vi "TestModule_Main.vi"() -> ()   [LabVIEW 2021]
uses:
  SubVI/TcpCmd_003/SubVI/SampleStatus.ctl
  SubVI/TcpCmd_003/SubVI/TcpCommunicationClientCMD.ctl
  SubVI/ErrorLogMode.ctl
  SubVI/MainStatus.ctl
panel:
  out "Message":string
  in  "SampleStatus":T1
  in  "Main Tab":enum32{"操作", "TCP"}(tab)
  out "TCPDataLog":T2(array[cluster])
  in  "Send Data":string
  in  "Send":bool
  out "ReadData":string
  in  "中央PCアドレス":string="192.168.0.1"
  in  "ポート":u16=8501
  out "TcpOK?":bool
  out "SettingFilePath":path
  in  "DataFilePath":path=path "Test_DataFile"
  out "SampleName":string
  in  "Quit":bool
  out "Quit?":bool
  # "Test Module Main"
  # "Ver. 0.01"
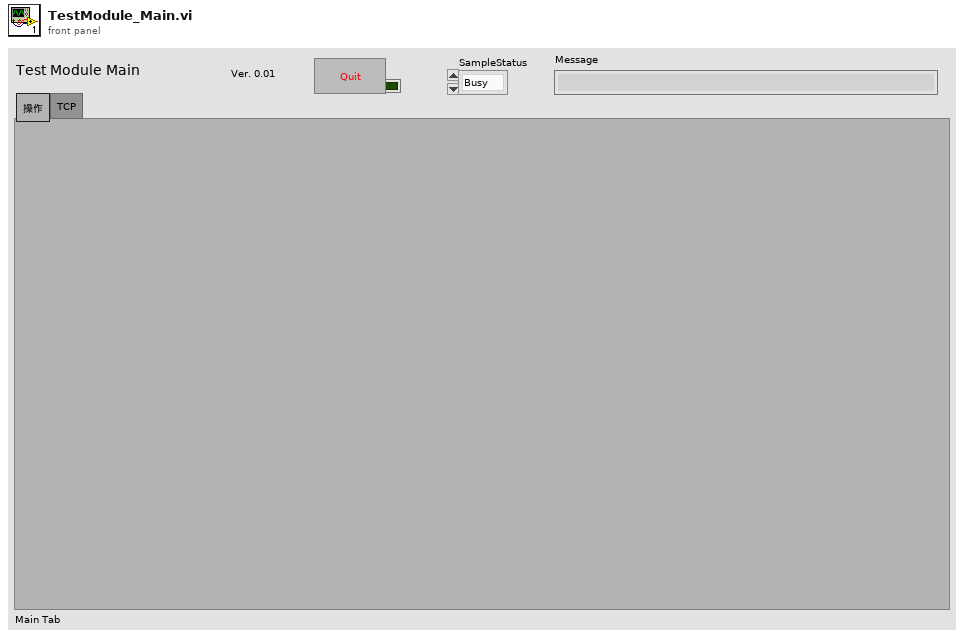
[diagram p1: front panel]
types:
  T1 = typedef "SampleStatus.ctl" = enum16{"Busy", "Ready", "Done", "Error"}
  T2 = cluster{"Command":string, "ReadData":string, "Send Data":string}[]
  T3 = typedef "TcpCommunicationClientCMD.ctl" = enum16{"Read", "Write", "Close"}
  T4 = typedef "ErrorLogMode.ctl" = enum16{"Init", "Add"}
  T5 = typedef "MainStatus.ctl" = enum16{"Init", "Status", "Placed", "Setting", "Start", "Data", "Collected", "Quit"}
  T6 = cluster{"Command":string, "ReadData":string, "t":string}
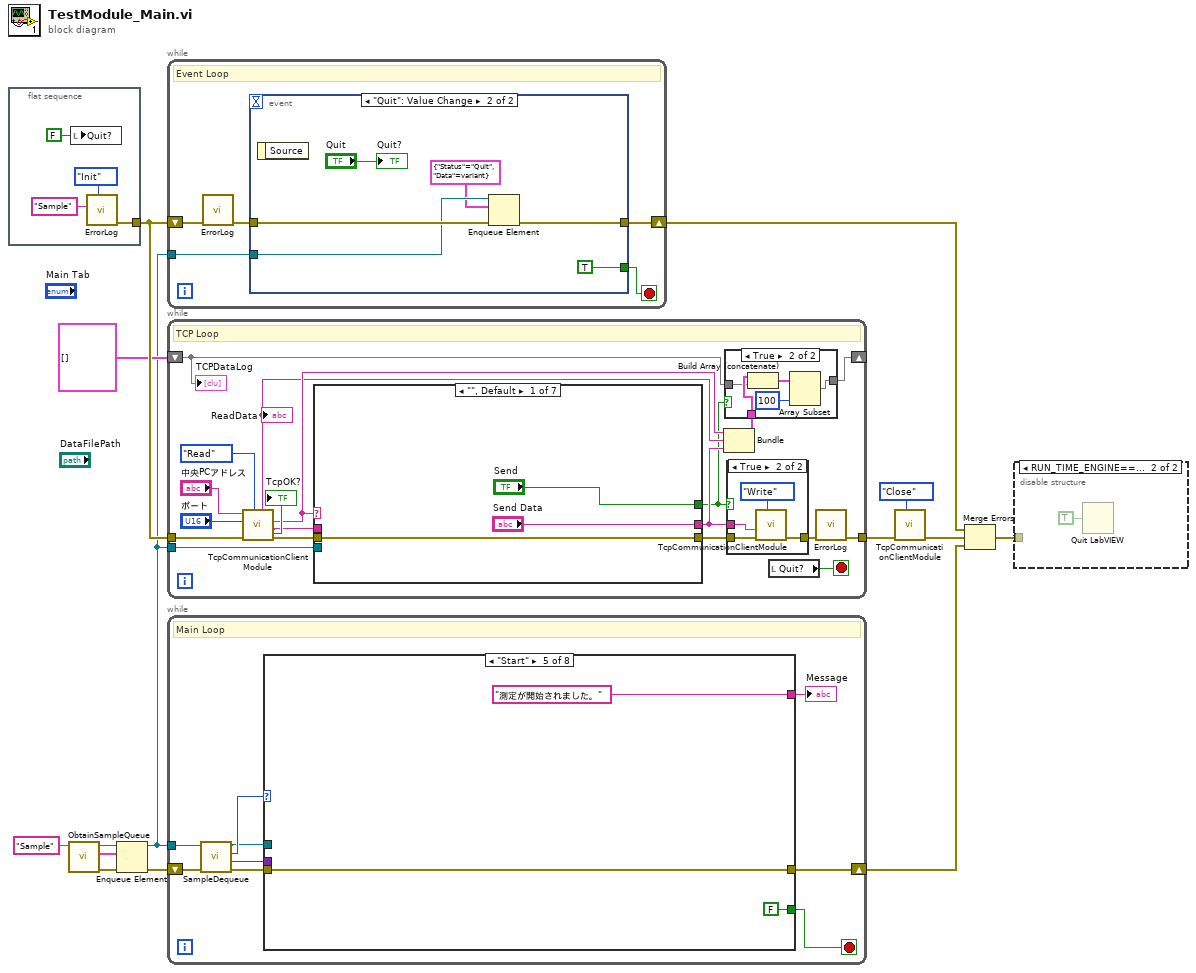
[diagram p0: block diagram]
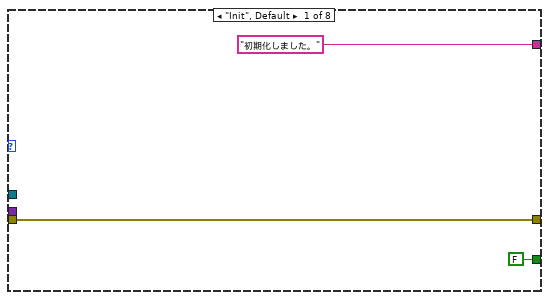
[diagram p3: hidden frame]
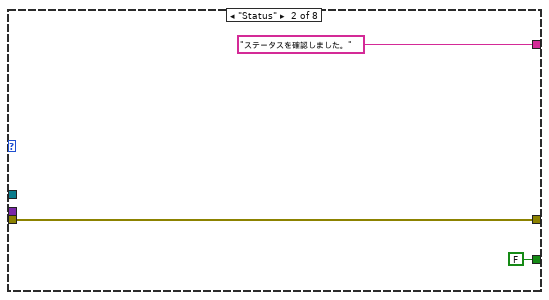
[diagram p4: hidden frame]
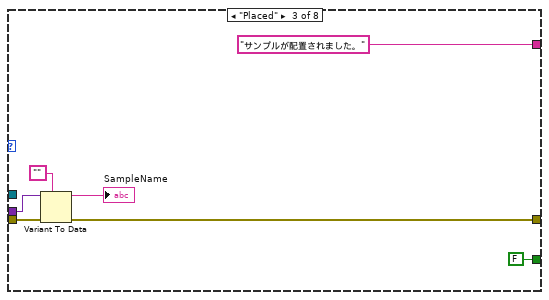
[diagram p5: hidden frame]
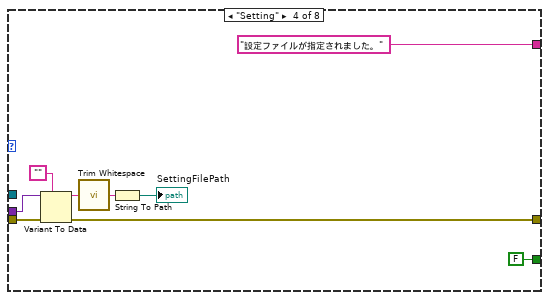
[diagram p6: hidden frame]
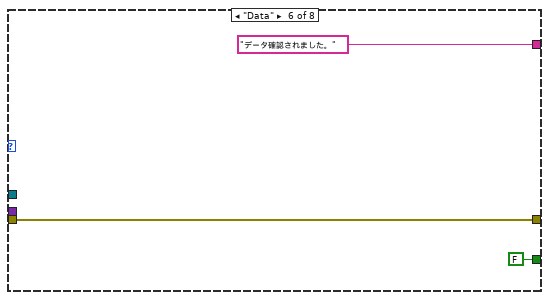
[diagram p7: hidden frame]
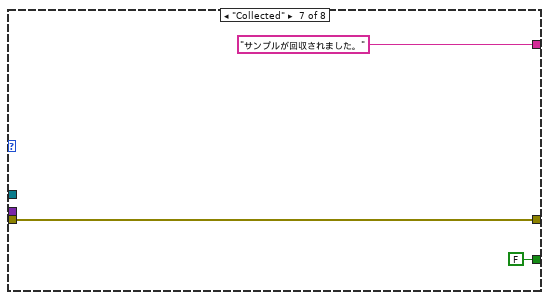
[diagram p8: hidden frame]
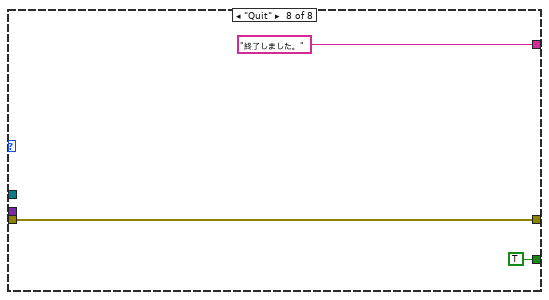
[diagram p9: hidden frame]
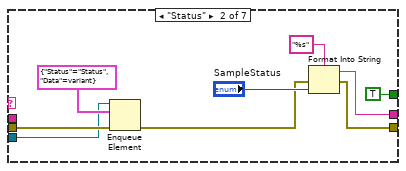
[diagram p12: hidden frame]
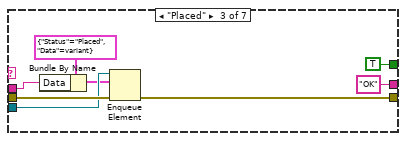
[diagram p13: hidden frame]
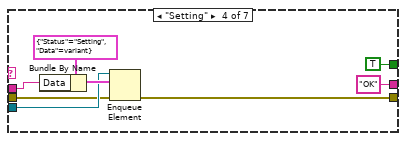
[diagram p14: hidden frame]
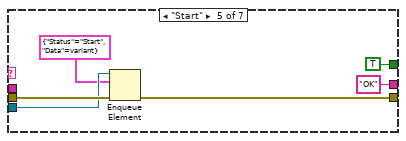
[diagram p15: hidden frame]
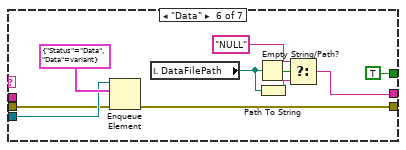
[diagram p16: hidden frame]
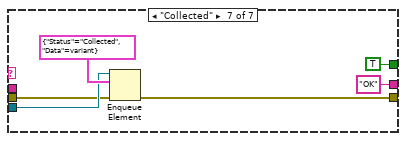
[diagram p17: hidden frame]
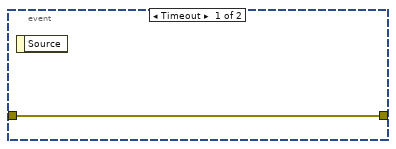
[diagram p18: hidden frame]
diagram:
  n1 = flat-sequence {
    tunnel: [w18] -> w14
    frame #0 {
      n2 = local write "Quit?"(FALSE ("Quit?")) -> ()
      n3 = call "ErrorLog.vi"("ErrorLogMode"=ErrorLogMode."Init", "ModuleName"="Sample") -> ("error out"=w18:errorcluster)  [unwired: 8 in, 1 out]
    }
  }
  n4 = call "ObtainSampleQueue.vi"("QName"="Sample") -> ("ErrorOut"=w10:errorcluster, "SampleQ"=w7:cluster{"Status":T5, "Data":variant}, "QueueOut"=w9:refnum<queue>)  [unwired: 8 in]
  n5 = Enqueue Element(queue=w9, element=w7, error in (no error)=w10) -> (queue out=w5:refnum<queue>, error out=w8:errorcluster)  [unwired: 1 in, 1 out]
  n6 = while {
    shift-right: [w21] -> w3
    shift-left: w14 -> [w22]
    tunnel: w5 -> [w19]
    stop <- w23 stop-if-true
    # "Event Loop"
    n7 = call "ErrorLog.vi"("error in (no error)"=w22) -> ("error out"=w20:errorcluster)  [unwired: 9 in, 1 out]
    n8 = event shown="[1] \"Quit\": Value Change" {
      selector: _ -> [_ _]
      dyn-events: _ -> [_ _]
      timeout: _ -> [_ _]
      tunnel: [_ TRUE] -> w23
      tunnel: [w24 w27] -> w21
      tunnel: w20 -> [w24 w28]
      tunnel: w19 -> [_ w26]
      event Timeout {
        n9 = event-data() -> ()  [unwired: 1 in, 1 out]
      }
      event "Quit": Value Change {
        n10 = event-data() -> ()  [unwired: 1 in, 1 out]
        n11 = Enqueue Element(queue=w26, element=cluster{"Status":T5, "Data":variant} {"Status"=enum."Quit", "Data"=variant}, error in (no error)=w28) -> (error out=w27:errorcluster)  [unwired: 1 in, 2 out]
        "Quit?" <- "Quit"
      }
    }
  }
  n12 = while {
    tunnel: w14 -> [w49]
    tunnel: [w43] -> w13
    shift-right: [w39] -> _
    shift-left: T2 [] -> [w35]
    tunnel: w5 -> [w31]
    stop <- w48 stop-if-true
    # "TCP Loop"
    n13 = call "TcpCommunicationClientModule.vi"("TcpCommunicationClientCMD"=TcpCommunicationClientCMD."Read", "エラー入力（エラーなし）"=w49, "ポート"="ポート", "アドレス"="中央PCアドレス") -> ("エラー出力"=w42:errorcluster, "Data"=w32:string, "Command"=w36:string, "TcpOK?"=→"TcpOK?":bool, "ReadData"=w34:string)  [unwired: 3 in]
    "ReadData" <- w34
    n14 = case shown="\"\", Default" w36 {
      tunnel: w42 -> [w63 w66 w77 w83 w92 w96 w106]
      tunnel: [w63 w71 w75 w81 w90 w95 w105] -> w41
      tunnel: ["Send Data" w70 "OK" ("Send Data") "OK" ("Send Data") "OK" ("Send Data") w99 "OK" ("t")] -> w37
      tunnel: ["Send" TRUE ("Send") TRUE ("Send") TRUE ("Send") TRUE ("Send") TRUE ("Send") TRUE ("Send")] -> w33
      tunnel: w32 -> [_ _ w73 w82 _ _ _]
      tunnel: w31 -> [_ w65 w76 w84 w91 w97 w107]
      frame "", Default {
      }
      frame "Status" {
        n15 = Enqueue Element(queue=w65, element=cluster{"Status":T5, "Data":variant} {"Status"=enum."Status", "Data"=variant}, error in (no error)=w66) -> (error out=w64:errorcluster)  [unwired: 1 in, 2 out]
        n16 = Format Into String(format string="%s" ("形式文字列"), error in=w64, "SampleStatus") -> (resulting string=w70:string, error out=w71:errorcluster)  [unwired: 1 in]
      }
      frame "Placed" {
        n17 = Bundle By Name(cluster=cluster{"Status":T5, "Data":variant} {"Status"=enum."Placed", "Data"=variant} ("element"), "Data"=w73) -> (w74:cluster{"Status":T5, "Data":variant})
        n18 = Enqueue Element(queue=w76, element=w74, error in (no error)=w77) -> (error out=w75:errorcluster)  [unwired: 1 in, 2 out]
      }
      frame "Setting" {
        n19 = Bundle By Name(cluster=cluster{"Status":T5, "Data":variant} {"Status"=enum."Setting", "Data"=variant} ("element"), "Data"=w82) -> (w85:cluster{"Status":T5, "Data":variant})
        n20 = Enqueue Element(queue=w84, element=w85, error in (no error)=w83) -> (error out=w81:errorcluster)  [unwired: 1 in, 2 out]
      }
      frame "Start" {
        n21 = Enqueue Element(queue=w91, element=cluster{"Status":T5, "Data":variant} {"Status"=enum."Start", "Data"=variant}, error in (no error)=w92) -> (error out=w90:errorcluster)  [unwired: 1 in, 2 out]
      }
      frame "Data" {
        n22 = Enqueue Element(queue=w97, element=cluster{"Status":T5, "Data":variant} {"Status"=enum."Data", "Data"=variant}, error in (no error)=w96) -> (error out=w95:errorcluster)  [unwired: 1 in, 2 out]
        n23 = local read "DataFilePath"() -> (w103:path)
        n24 = Empty String/Path?(string/path=w103) -> (empty?=w101:bool)
        n25 = Path To String(path=w103) -> (string=w102:string)
        n26 = Select(t="NULL", s=w101, f=w102) -> (s? t:f=w99:string)
      }
      frame "Collected" {
        n27 = Enqueue Element(queue=w107, element=cluster{"Status":T5, "Data":variant} {"Status"=enum."Collected", "Data"=variant}, error in (no error)=w106) -> (error out=w105:errorcluster)  [unwired: 1 in, 2 out]
      }
    }
    n28 = Bundle("Command"=w36, "ReadData"=w34, "t"=w37) -> (w38:T6)  [unwired: 1 in]
    n29 = case shown="True" w33 {
      tunnel: [w50 w52] -> w39
      tunnel: w38 -> [_ w54]
      tunnel: w35 -> [w50 w53]
      frame False {
      }
      frame True {
        n30 = Build Array (concatenate)(w54, w53) -> (w55:T2)
        n31 = Array Subset(array=w55, length=100 ("長さ")) -> (w52:T2)  [unwired: 1 in]
      }
    }
    n32 = case shown="True" w33 {
      tunnel: w41 -> [w56 w59]
      tunnel: [w56 w58] -> w40
      tunnel: w37 -> [_ w57]
      frame False {
      }
      frame True {
        n33 = call "TcpCommunicationClientModule.vi"("TcpCommunicationClientCMD"=TcpCommunicationClientCMD."Write", "エラー入力（エラーなし）"=w59, "WriteData"=w57) -> ("エラー出力"=w58:errorcluster)  [unwired: 4 in, 4 out]
      }
    }
    n34 = local read "Quit?"() -> (w48:bool)
    n35 = call "ErrorLog.vi"("error in (no error)"=w40) -> ("error out"=w43:errorcluster)  [unwired: 9 in, 1 out]
    "TCPDataLog" <- w35
  }
  n36 = while {
    tunnel: w5 -> [w118]
    shift-right: [w113] -> w2
    shift-left: w8 -> [w119]
    stop <- w112 stop-if-true
    # "Main Loop"
    n37 = call "SampleDequeue.vi"("エラー入力（エラーなし）"=w119, "キュー入力"=w118) -> ("エラー出力"=w116:errorcluster, "Data"=w114:variant, "StepName"=w117:T5, "キュー出力"=w115:refnum<queue>)  [unwired: 6 in]
    n38 = case shown="\"Start\"" w117 {
      tunnel: w116 -> [w122 w125 w130 w139 w142 w145 w148 w153]
      tunnel: w115 -> [_ _ _ _ _ _ _ _]
      tunnel: w114 -> [_ _ w128 w137 _ _ _ _]
      tunnel: [w122 w125 w129 w138 w142 w145 w148 w153] -> w113
      tunnel: [FALSE FALSE FALSE FALSE FALSE FALSE FALSE TRUE] -> w112
      tunnel: ["初期化しました。" "ステータスを確認しました。" "サンプルが配置されました。" "設定ファイルが指定されました。" "測定が開始されました。" "データ確認されました。" "サンプルが回収されました。" "終了しました。"] -> w111
      frame "Init", Default {
      }
      frame "Status" {
      }
      frame "Placed" {
        n39 = Variant To Data(error in=w130, type="", Variant=w128) -> (data=→"SampleName":string, error out=w129:errorcluster)
      }
      frame "Setting" {
        n40 = Variant To Data(error in=w139, type="", Variant=w137) -> (data=w133:string, error out=w138:errorcluster)
        n41 = call <vilib>:"Trim Whitespace.vi"("string"=w133) -> ("trimmed string"=w135:string)  [unwired: 1 in]
        n42 = String To Path(string=w135) -> (path=→"SettingFilePath":path)
      }
      frame "Start" {
      }
      frame "Data" {
      }
      frame "Collected" {
      }
      frame "Quit" {
      }
    }
    "Message" <- w111
  }
  n43 = call "TcpCommunicationClientModule.vi"("TcpCommunicationClientCMD"=TcpCommunicationClientCMD."Close", "エラー入力（エラーなし）"=w13) -> ("エラー出力"=w4:errorcluster)  [unwired: 5 in, 4 out]
  n44 = Merge Errors(w3, w4, w2) -> (w1:errorcluster)
  n45 = disable-structure shown="RUN_TIME_ENGINE==True" {
    disable-tunnel: w1 -> [_ _]
    frame condition #0 (active) {
    }
    frame condition #1 {
      n46 = Quit LabVIEW(quit? (T)=TRUE) -> ()
    }
  }
